vi "EvaluateOneRow.vi"(8 "Error In":errorcluster, 11 "OneString":string="dbcfg fgd bdegcaf fgec aegbdf ecdfab fbedc dacgb gdcebf gf | cefg dcbef fcge gbcadfe") -> (0 "Error Out":errorcluster, 3 "number":i32=4948)   [LabVIEW 2020, in "2021_8.lvclass"]
uses:
  2021_8.lvclass
  6650c231-ec79-43c6-a03f-3b69b835ea87.vi
  b0ebf4ca-cbf1-4ce0-92b1-cda46eb14d0c.vi
  f1bdf902-0adb-4505-a830-97cba88f444f.vi
  5bd7c106-27c0-4e97-a852-251e1e95a34d.vi
  118c3635-3ba3-46eb-8919-0376fe602ad3.vi
  31264f6e-4644-4268-8b29-d530524c077c.vi
  1517e18e-c622-44f4-9be2-471113a16f81.vi
  ccff8709-7a9d-4d3b-b9c5-f645e1f7c142.vi
  895731a1-4916-48ec-9da7-2ffc94040f8c.vi
  7a22b7fc-ffc8-42fa-bd17-9a4c3744b480.vi
  fee79420-5269-48e8-b4f2-c0721e77aa49.vi
  7e0e2c57-2e26-422c-b2e4-656288a5e421.vi
  6650c231-ec79-43c6-a03f-3b69b835ea87.vi/be6f088c-3e4b-4523-ad48-2cdc85bad38a.vi
  6650c231-ec79-43c6-a03f-3b69b835ea87.vi/f202eadf-433e-4cdb-b986-b2351ce8d73c.vi
  6650c231-ec79-43c6-a03f-3b69b835ea87.vi/094751bc-bcf2-4346-afae-53942128b536.vi
  6650c231-ec79-43c6-a03f-3b69b835ea87.vi/06ee343e-764f-4086-89d5-f578778d243c.vi
  5bd7c106-27c0-4e97-a852-251e1e95a34d.vi/be6f088c-3e4b-4523-ad48-2cdc85bad38a.vi
  5bd7c106-27c0-4e97-a852-251e1e95a34d.vi/f202eadf-433e-4cdb-b986-b2351ce8d73c.vi
  5bd7c106-27c0-4e97-a852-251e1e95a34d.vi/094751bc-bcf2-4346-afae-53942128b536.vi
  5bd7c106-27c0-4e97-a852-251e1e95a34d.vi/06ee343e-764f-4086-89d5-f578778d243c.vi
  ccff8709-7a9d-4d3b-b9c5-f645e1f7c142.vi/be6f088c-3e4b-4523-ad48-2cdc85bad38a.vi
  ccff8709-7a9d-4d3b-b9c5-f645e1f7c142.vi/f202eadf-433e-4cdb-b986-b2351ce8d73c.vi
  ccff8709-7a9d-4d3b-b9c5-f645e1f7c142.vi/094751bc-bcf2-4346-afae-53942128b536.vi
  ccff8709-7a9d-4d3b-b9c5-f645e1f7c142.vi/06ee343e-764f-4086-89d5-f578778d243c.vi
  fee79420-5269-48e8-b4f2-c0721e77aa49.vi/be6f088c-3e4b-4523-ad48-2cdc85bad38a.vi
  fee79420-5269-48e8-b4f2-c0721e77aa49.vi/f202eadf-433e-4cdb-b986-b2351ce8d73c.vi
  fee79420-5269-48e8-b4f2-c0721e77aa49.vi/094751bc-bcf2-4346-afae-53942128b536.vi
  7e0e2c57-2e26-422c-b2e4-656288a5e421.vi/be6f088c-3e4b-4523-ad48-2cdc85bad38a.vi
  7e0e2c57-2e26-422c-b2e4-656288a5e421.vi/f202eadf-433e-4cdb-b986-b2351ce8d73c.vi
  7e0e2c57-2e26-422c-b2e4-656288a5e421.vi/094751bc-bcf2-4346-afae-53942128b536.vi
  7e0e2c57-2e26-422c-b2e4-656288a5e421.vi/06ee343e-764f-4086-89d5-f578778d243c.vi
panel:
  out "Segemtns":string[](array[string])=["d", "", "g", "", "", "f", ""]
  out "Array":string[](array[string])=["aegbdf", "gf", "dacgb", "dbcfg", "fgec", "dbcfg", "ecdfab", "fgd", "bdegcaf", "gdcebf"]
  # "#5"
  # "#5"
  # "#8"
  # "#4"
  # "#6"
  # "#6"
  # "#5"
  # "#5"
  # "#6"
  # "#2"
  # "7"
  # "1"
  # "8"
  # "4"
  # "3"
  # "6"
  # "2"
  # "5"
  # "0"
  # "1"
  # "2"
  # "3: fOR ALL #5 CHECK THAT &'S sEGMENT ALL EXISTS\n6: WHen 1's Segemtn only macthes one\n2: 5 segments (and not 3/found) and not hace lower right segment"
  # "3"
  # "4"
  # "5"
  # "6"
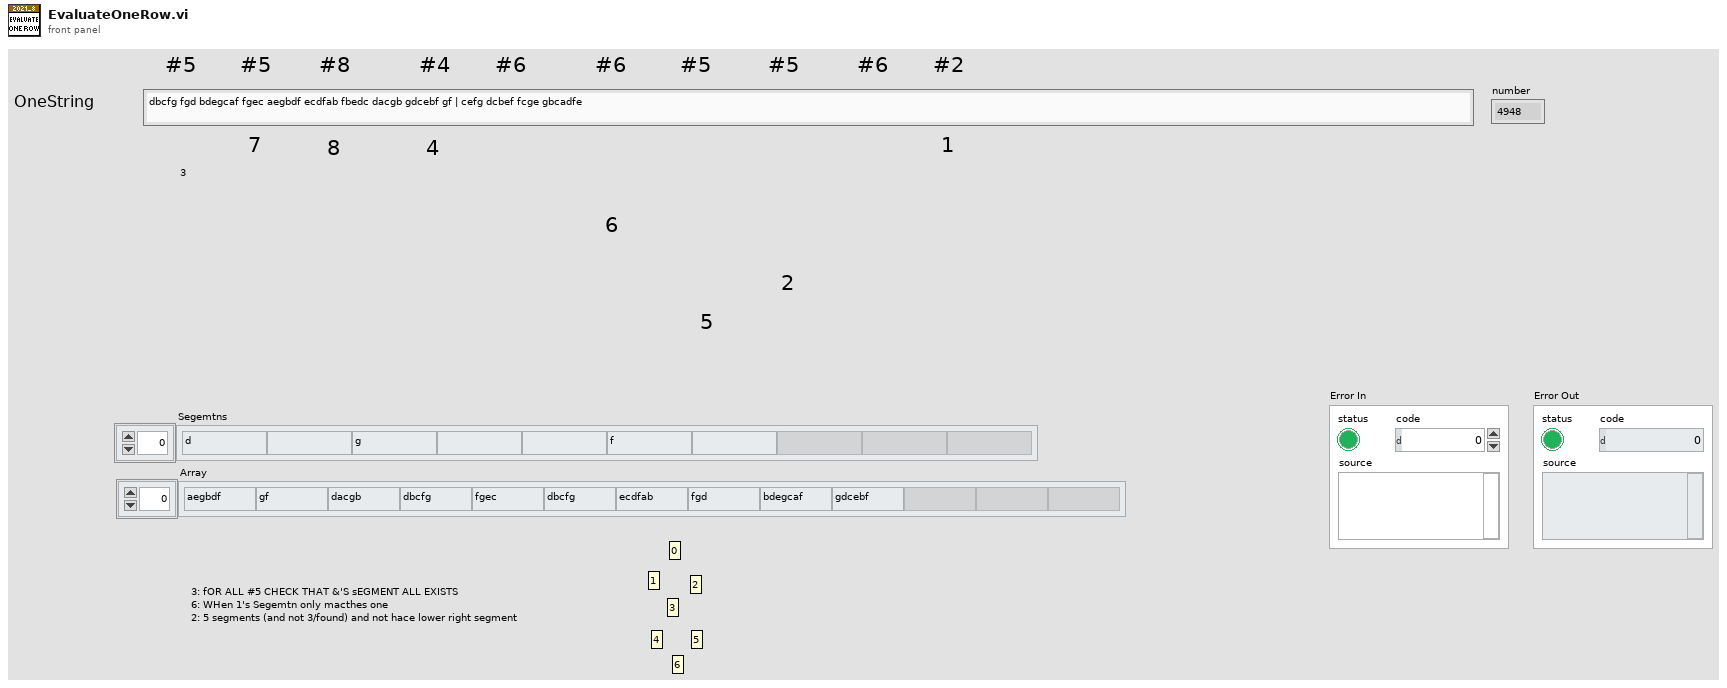
[diagram p1: front panel]
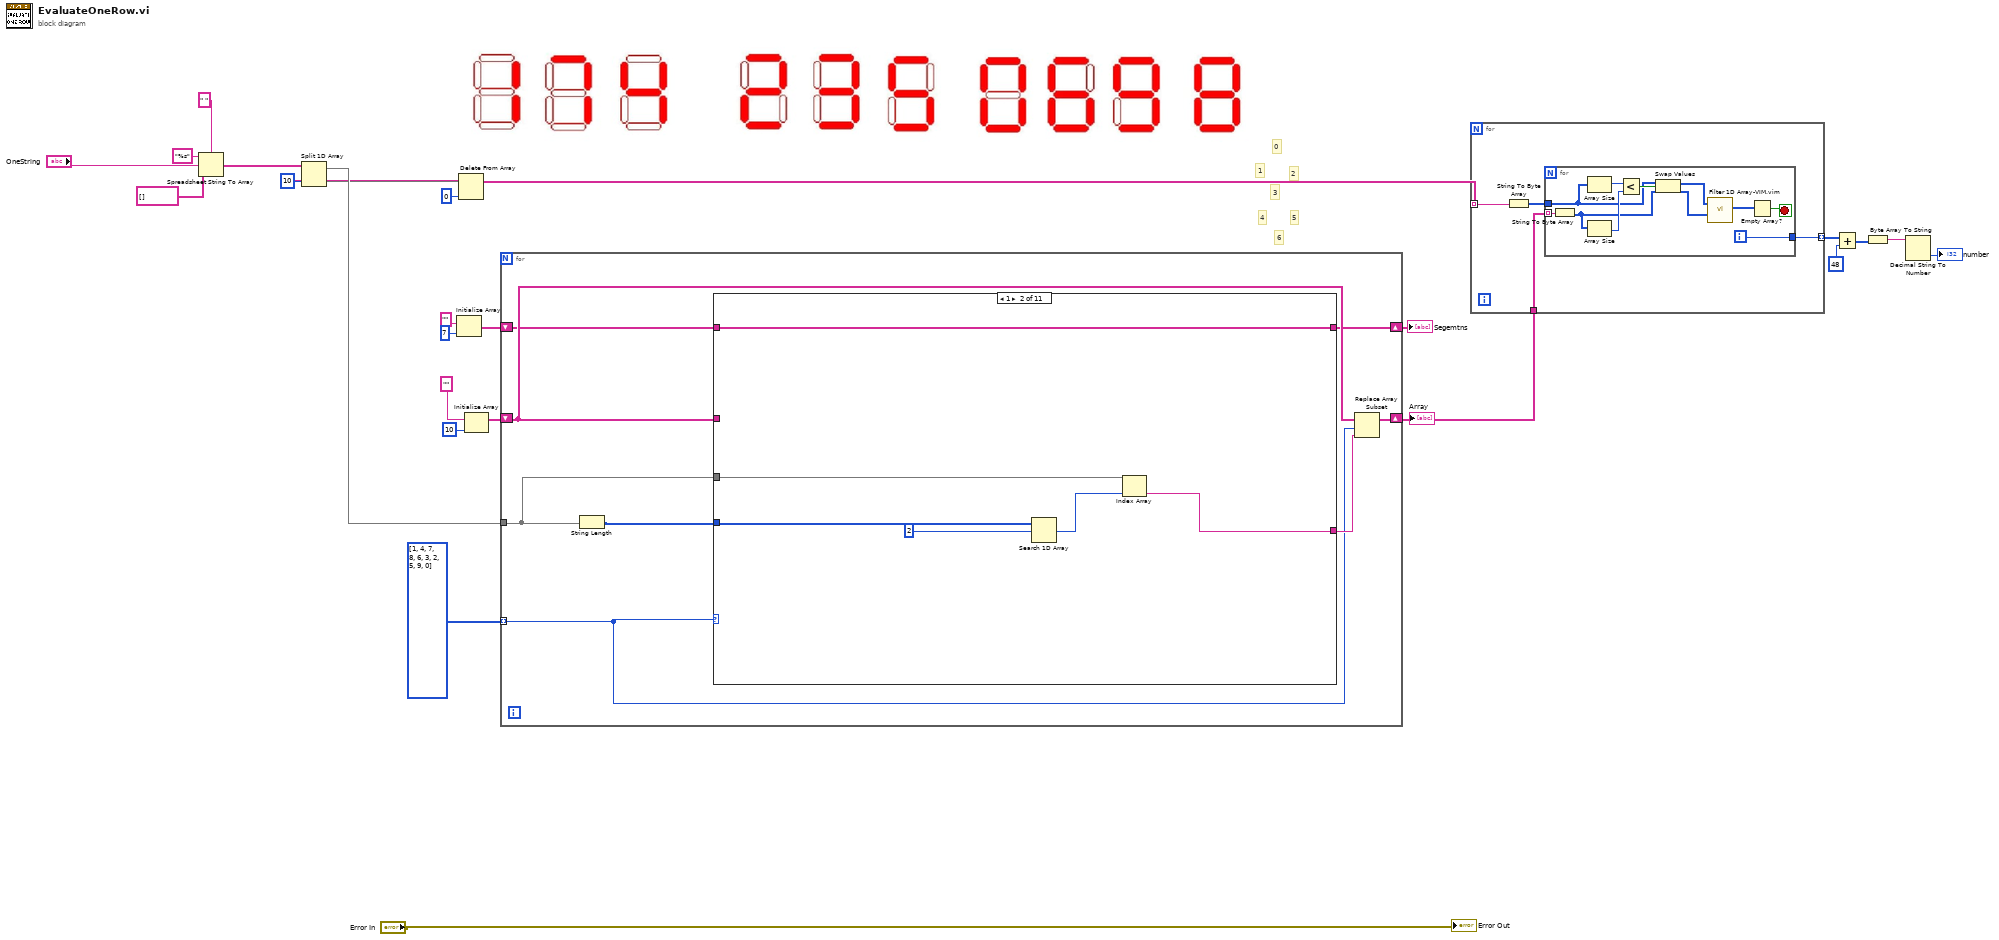
[diagram p0: block diagram]
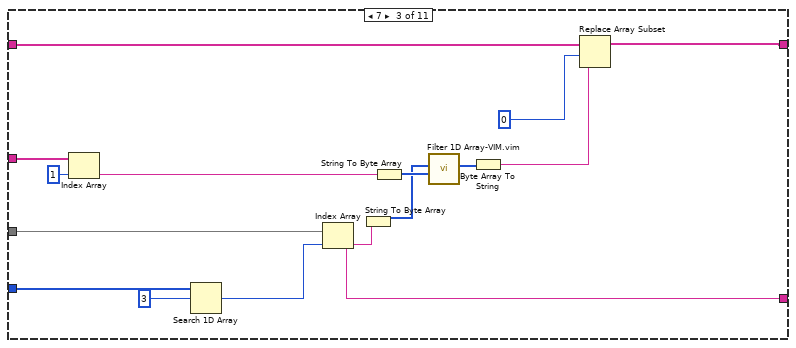
[diagram p3: hidden frame]
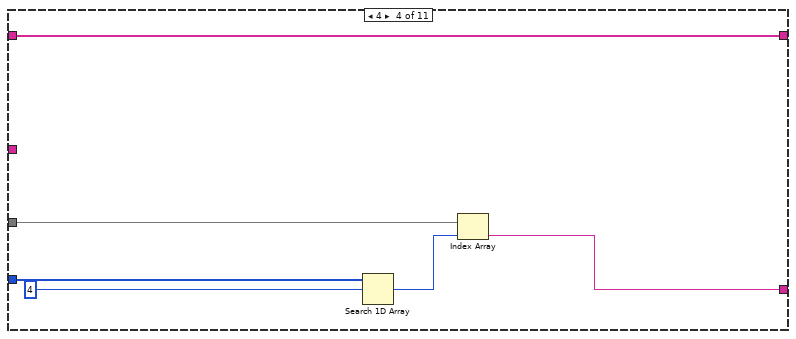
[diagram p4: hidden frame]
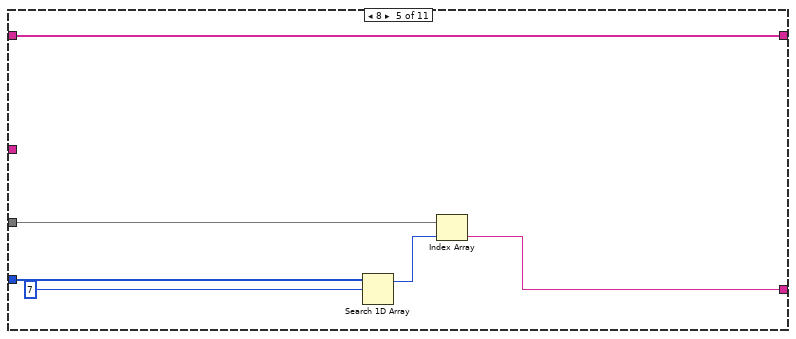
[diagram p5: hidden frame]
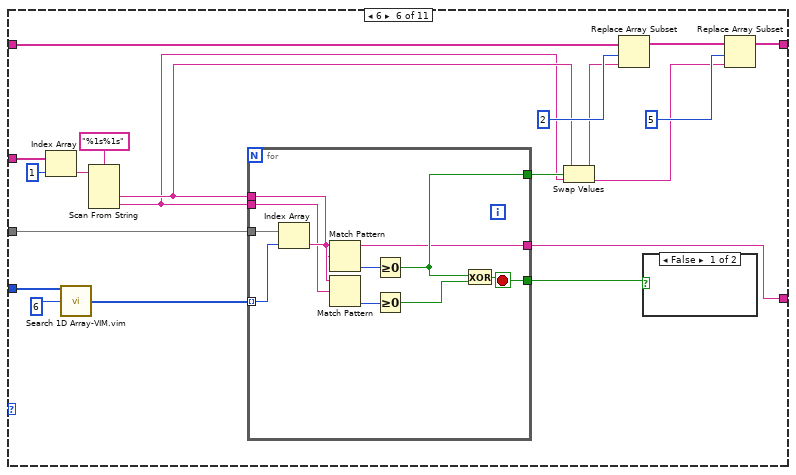
[diagram p6: hidden frame]
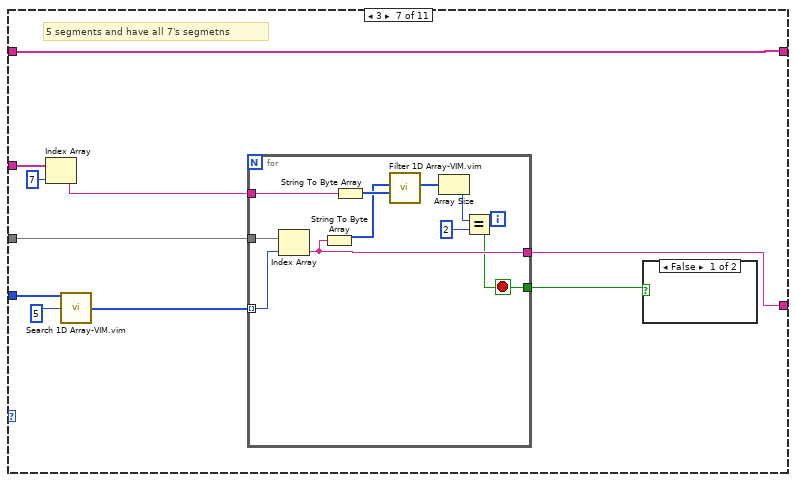
[diagram p8: hidden frame]
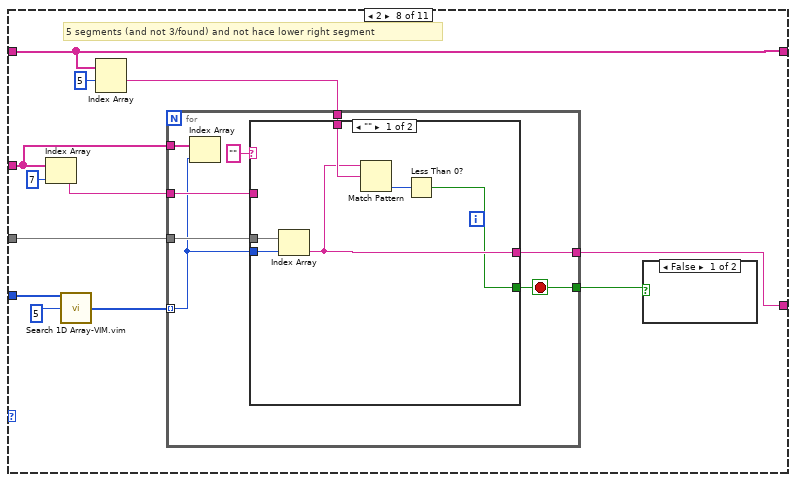
[diagram p10: hidden frame]
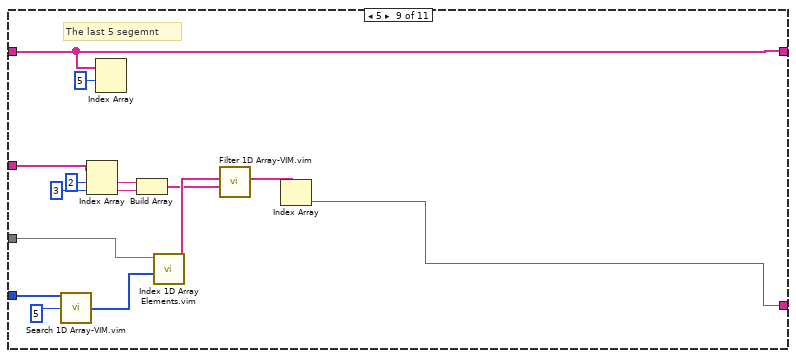
[diagram p13: hidden frame]
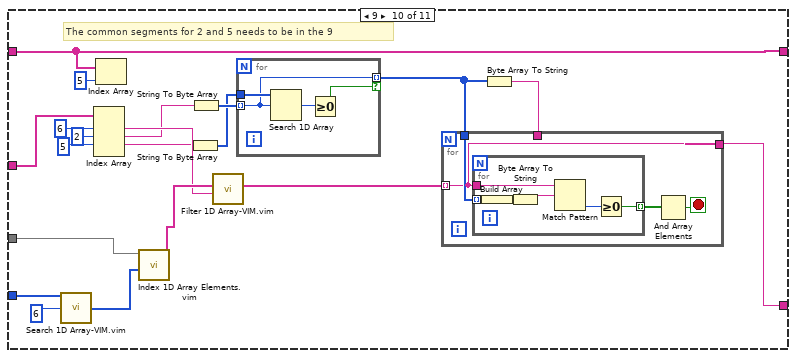
[diagram p14: hidden frame]
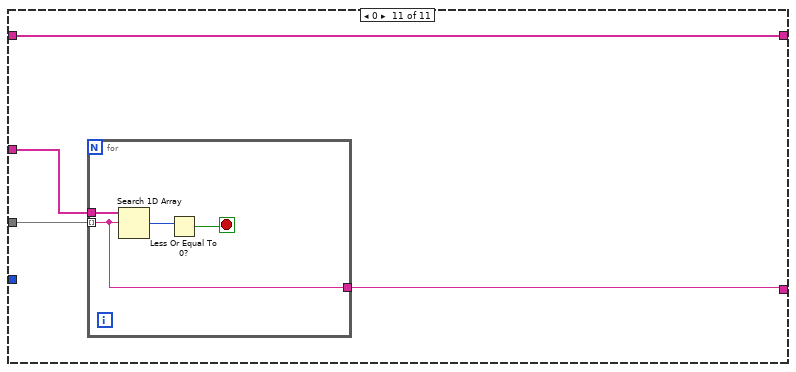
[diagram p15: hidden frame]
diagram:
  # "6"
  # "5"
  # "4"
  # "3"
  # "2"
  # "1"
  # "0"
  n1 = Spreadsheet String To Array(delimiter (Tab)=" ", format string="%s", spreadsheet string="OneString", array type (2D Dbl)=string[] []) -> (array=w21:string[])
  n2 = Split 1D Array(array=w21, index=10) -> (first subarray=w18:string[], second subarray=w5:string[])
  n3 = Initialize Array("", 7 ("dimension size")) -> (w14:string[])
  n4 = Delete From Array(array=w5, index=0) -> (array with subset deleted=w4:string[])  [unwired: 1 in, 1 out]
  n5 = Initialize Array("", 10 ("dimension size")) -> (w17:string[])
  n6 = for {
    tunnel: w18 -> [w28]
    shift-right: [w30] -> w10
    shift-left: w17 -> [w33]
    tunnel: i32[] [1, 4, 7, 8, 6, 3, 2, 5, 9, 0] -> [w29] mode=indexing
    shift-right: [w26] -> w11
    shift-left: w14 -> [w27]
    n7 = String Length(string=w28) -> (length=w32:i32[])
    n8 = case shown="1" w29 {
      tunnel: w33 -> [_ _ w51 _ _ w84 w104 w119 w151 w174 w194]
      tunnel: w32 -> [_ w40 w55 w61 w67 w87 w107 w129 w158 w178 _]
      tunnel: [_ w35 w48 w56 w62 w76 w100 w123 w144 w163 w193] -> w31
      tunnel: w28 -> [_ w37 w53 w58 w64 w82 w102 w125 w153 w172 w195]
      tunnel: w27 -> [w34 w38 w44 w59 w65 w80 w99 w121 w156 w176 w196]
      tunnel: [w34 w38 w43 w59 w65 w73 w99 w121 w156 w176 w196] -> w26
      frame Default {
      }
      frame 1 {
        n9 = Search 1D Array(1D array=w40, element=2) -> (index of element=w36:i32)  [unwired: 1 in]
        n10 = Index Array(array=w37, index=w36) -> (element=w35:string)
      }
      frame 7 {
        n11 = Index Array(array=w51, index=1) -> (element=w49:string)
        n12 = Search 1D Array(1D array=w55, element=3) -> (index of element=w52:i32)  [unwired: 1 in]
        n13 = Index Array(array=w53, index=w52) -> (element=w48:string)
        n14 = String To Byte Array(string=w48) -> (unsigned byte array=w46:u8[])
        n15 = String To Byte Array(string=w49) -> (unsigned byte array=w47:u8[])
        n16 = call "Filter 1D Array-VIM.vim"("Item(s) to Filter"=w47, "Array"=w46) -> ("Filtered Array"=w45:u8[])  [unwired: 5 in, 1 out]
        n17 = Byte Array To String(unsigned byte array=w45) -> (string=w41:string)
        n18 = Replace Array Subset(array=w44, new element=w41, index=0) -> (w43:string[])
      }
      frame 4 {
        n19 = Search 1D Array(1D array=w61, element=4) -> (index of element=w57:i32)  [unwired: 1 in]
        n20 = Index Array(array=w58, index=w57) -> (element=w56:string)
      }
      frame 8 {
        n21 = Search 1D Array(1D array=w67, element=7) -> (index of element=w63:i32)  [unwired: 1 in]
        n22 = Index Array(array=w64, index=w63) -> (element=w62:string)
      }
      frame 6 {
        n23 = Index Array(array=w84, index=1) -> (element=w78:string)
        n24 = call "Search 1D Array-VIM.vim"("Array"=w87, "Element Data"=6) -> ("Indices of Elements"=w85:i32[])  [unwired: 7 in]
        n25 = Scan From String(format string="%1s%1s", input string=w78) -> (output 1=w69:string, output 2=w68:string)  [unwired: 4 in, 3 out]
        n26 = for {
          tunnel: w85 -> [w95] mode=indexing
          tunnel: w82 -> [w97]
          tunnel: [w96] -> w81
          tunnel: w69 -> [w88]
          tunnel: w68 -> [w89]
          tunnel: [w90] -> w76
          tunnel: [w91] -> w75
          stop <- w96 stop-if-true
          n27 = Index Array(array=w97, index=w95) -> (element=w90:string)
          n28 = Match Pattern(string=w90, regular expression=w88) -> (offset past match=w94:i32)  [unwired: 1 in, 3 out]
          n29 = Match Pattern(string=w90, regular expression=w89) -> (offset past match=w93:i32)  [unwired: 1 in, 3 out]
          n30 = Greater Or Equal To 0?(x=w94) -> (x >= 0?=w91:bool)
          n31 = Greater Or Equal To 0?(x=w93) -> (x >= 0?=w92:bool)
          n32 = Exclusive Or(1:w92, 2:w91) -> (0:w96:bool)
        }
        n33 = Swap Values(12:w69, 13:w75, 14:w68) -> (1:w71:string, 3:w70:string)
        n34 = Replace Array Subset(array=w80, new element=w71, index=2) -> (w74:string[])
        n35 = case shown="False" w81 {
          frame False {
          }
          frame True {
          }
        }
        n36 = Replace Array Subset(array=w74, new element=w70, index=5) -> (w73:string[])
      }
      frame 3 {
        # "5 segments and have all 7's segmetns"
        n37 = Index Array(array=w104, index=7) -> (element=w98:string)
        n38 = call "Search 1D Array-VIM.vim"("Array"=w107, "Element Data"=5) -> ("Indices of Elements"=w105:i32[])  [unwired: 7 in]
        n39 = for {
          tunnel: w105 -> [w116] mode=indexing
          tunnel: w102 -> [w117]
          tunnel: [w108] -> w101
          tunnel: [w113] -> w100
          tunnel: w98 -> [w112]
          stop <- w108 stop-if-true
          n40 = Index Array(array=w117, index=w116) -> (element=w113:string)
          n41 = String To Byte Array(string=w113) -> (unsigned byte array=w114:u8[])
          n42 = String To Byte Array(string=w112) -> (unsigned byte array=w115:u8[])
          n43 = call "Filter 1D Array-VIM.vim"("Item(s) to Filter"=w115, "Array"=w114) -> ("Filtered Array"=w111:u8[])  [unwired: 5 in, 1 out]
          n44 = Array Size(array=w111) -> (size(s)=w110:i32)
          n45 = Equal?(x=w110, y=2) -> (x = y?=w108:bool)
        }
        n46 = case shown="False" w101 {
          frame False {
          }
          frame True {
          }
        }
      }
      frame 2 {
        # "5 segments (and not 3/found) and not hace lower right segment"
        n47 = Index Array(array=w119, index=7) -> (element=w122:string)
        n48 = call "Search 1D Array-VIM.vim"("Array"=w129, "Element Data"=5) -> ("Indices of Elements"=w127:i32[])  [unwired: 7 in]
        n49 = Index Array(array=w121, index #1=5 ("index")) -> (element #1=w118:string)  [unwired: 1 in, 1 out]
        n50 = for {
          tunnel: w127 -> [w132] mode=indexing
          tunnel: w125 -> [w137]
          tunnel: [w134] -> w124
          tunnel: [w136] -> w123
          tunnel: w122 -> [w135]
          tunnel: w119 -> [w133]
          tunnel: w118 -> [w131]
          stop <- w134 stop-if-true
          n51 = Index Array(array=w133, index=w132) -> ()  [unwired: 1 out]
          n52 = case shown="\"\"" "" {
            tunnel: w137 -> [w143 _]
            tunnel: [w139 _] -> w136
            tunnel: w135 -> [_ _]
            tunnel: [w138 _] -> w134
            tunnel: w132 -> [w142 _]
            tunnel: w131 -> [w140 _]
            frame "" {
              n53 = Index Array(array=w143, index=w142) -> (element=w139:string)
              n54 = Match Pattern(string=w139, regular expression=w140) -> (offset past match=w141:i32)  [unwired: 1 in, 3 out]
              n55 = Less Than 0?(x=w141) -> (x < 0?=w138:bool)
            }
            frame Default {
            }
          }
        }
        n56 = case shown="False" w124 {
          frame False {
          }
          frame True {
          }
        }
      }
      frame 5 {
        # "The last 5 segemnt"
        n57 = call "Search 1D Array-VIM.vim"("Array"=w158, "Element Data"=5) -> ("Indices of Elements"=w152:i32[])  [unwired: 7 in]
        n58 = Index Array(array=w151, index #1=2 ("index"), index #2=3 ("index")) -> (element #1=w148:string, element #2=w147:string)
        n59 = Index Array(array=w156, index #1=5 ("index")) -> ()  [unwired: 1 in, 2 out]
        n60 = Build Array(w148, w147) -> (w145:string[])
        n61 = call "Index 1D Array Elements.vim"("indices"=w152, "array"=w153) -> ("elements"=w146:string[])  [unwired: 9 in]
        n62 = call "Filter 1D Array-VIM.vim"("Item(s) to Filter"=w145, "Array"=w146) -> ("Filtered Array"=w154:string[])  [unwired: 5 in, 1 out]
        n63 = Index Array(array=w154) -> (element=w144:string)  [unwired: 1 in]
      }
      frame 9 {
        # "The common segments for 2 and 5 needs to be in the 9"
        n64 = call "Search 1D Array-VIM.vim"("Array"=w178, "Element Data"=6) -> ("Indices of Elements"=w171:i32[])  [unwired: 7 in]
        n65 = Index Array(array=w174, index #1=6 ("index"), index #2=2 ("index"), index #3=5 ("index")) -> (element #1=w169:string, element #2=w166:string, element #3=w165:string)  [unwired: 1 in, 1 out]
        n66 = Index Array(array=w176, index=5) -> ()  [unwired: 1 out]
        n67 = call "Index 1D Array Elements.vim"("indices"=w171, "array"=w172) -> ("elements"=w170:string[])  [unwired: 9 in]
        n68 = String To Byte Array(string=w165) -> (unsigned byte array=w160:u8[])
        n69 = String To Byte Array(string=w166) -> (unsigned byte array=w161:u8[])
        n70 = call "Filter 1D Array-VIM.vim"("Item(s) to Filter"=w169, "Array"=w170) -> ("Filtered Array"=w164:string[])  [unwired: 5 in, 1 out]
        n71 = for {
          tunnel: w161 -> [w180] mode=indexing
          tunnel: w160 -> [w182]
          tunnel: [w180] -> w159 mode=indexing if=w179
          n72 = Search 1D Array(1D array=w182, element=w180) -> (index of element=w181:i32)  [unwired: 1 in]
          n73 = Greater Or Equal To 0?(x=w181) -> (x >= 0?=w179:bool)
        }
        n74 = Byte Array To String(unsigned byte array=w159) -> (string=w162:string)
        n75 = for {
          tunnel: w164 -> [w183] mode=indexing
          tunnel: w159 -> [w186]
          tunnel: [w183] -> w163
          tunnel: w162 -> [_]
          stop <- w184 stop-if-true
          n76 = for {
            tunnel: w183 -> [w192]
            tunnel: w186 -> [w191] mode=indexing
            tunnel: [w187] -> w185 mode=indexing
            n77 = Build Array(w191) -> (w190:u8[])
            n78 = Byte Array To String(unsigned byte array=w190) -> (string=w189:string)
            n79 = Match Pattern(string=w192, regular expression=w189) -> (offset past match=w188:i32)  [unwired: 1 in, 3 out]
            n80 = Greater Or Equal To 0?(x=w188) -> (x >= 0?=w187:bool)
          }
          n81 = And Array Elements(Boolean array=w185) -> (logical AND=w184:bool)
        }
      }
      frame 0 {
        n82 = for {
          tunnel: w195 -> [w197] mode=indexing
          tunnel: w194 -> [w200]
          tunnel: [w197] -> w193
          stop <- w198 stop-if-true
          n83 = Search 1D Array(1D array=w200, element=w197) -> (index of element=w199:i32)  [unwired: 1 in]
          n84 = Less Or Equal To 0?(x=w199) -> (x <= 0?=w198:bool)
        }
      }
    }
    n85 = Replace Array Subset(array=w33, new element=w31, index=w29) -> (w30:string[])
  }
  "Array" <- w10
  "Segemtns" <- w11
  n86 = for {
    tunnel: w4 -> [w204] mode=indexing
    tunnel: w10 -> [w202]
    tunnel: [w201] -> w9 mode=indexing
    n87 = String To Byte Array(string=w204) -> (unsigned byte array=w203:u8[])
    n88 = for {
      tunnel: w203 -> [w206]
      tunnel: w202 -> [w215] mode=indexing
      tunnel: [w212] -> w201
      i -> [w212]
      stop <- w213 stop-if-true
      n89 = String To Byte Array(string=w215) -> (unsigned byte array=w208:u8[])
      n90 = Array Size(array=w206) -> (size(s)=w211:i32)
      n91 = Array Size(array=w208) -> (size(s)=w210:i32)
      n92 = Less?(x=w211, y=w210) -> (x < y?=w209:bool)
      n93 = Swap Values(12:w206, 13:w209, 14:w208) -> (1:w207:u8[], 3:w205:u8[])
      n94 = call "Filter 1D Array-VIM.vim"("Item(s) to Filter"=w205, "Array"=w207) -> ("Filtered Array"=w214:u8[])  [unwired: 5 in, 1 out]
      n95 = Empty Array?(array=w214) -> (empty?=w213:bool)
    }
  }
  n96 = Add(x=w9, y=48 ("index")) -> (x+y=w7:i32[])
  n97 = Byte Array To String(unsigned byte array=w7) -> (string=w3:string)
  n98 = Decimal String To Number(string=w3) -> (number=→"number":i32)  [unwired: 2 in, 1 out]
  "Error Out" <- "Error In"
